vi "Write queue ref.vi"(10 "queue ref":refnum<queue>, 11 "Log Sinks in":refnum<class "Log Sinks.lvclass">) -> (3 "Log Sinks out":refnum<class "Log Sinks.lvclass">)   [LabVIEW 2019, in "TSC Event Logger.lvlib" / "Log Sinks.lvclass"]
uses:
  Log Sinks.lvclass
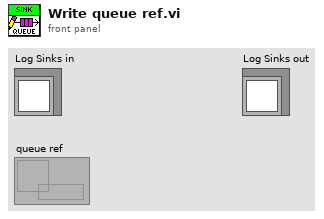
[diagram p1: front panel]
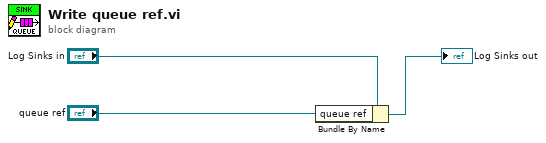
[diagram p0: block diagram]
diagram:
  n1 = Bundle By Name(cluster="Log Sinks in", "queue ref"="queue ref") -> (→"Log Sinks out":refnum<class "Log Sinks.lvclass">)
